vi "Invertor rate calc.vi"(6 "PID gains":T1={"proportional gain (Kc)"=60.0, "integral time (Ti, min)"=0.2, "derivative time (Td, min)"=0.0}, 7 "Output range":cluster{"output high":dbl, "output low":dbl}={"output high"=100.0, "output low"=0.0} {"output low" format="%.2f"; "output high" format="%.2f"}, 9 "V Max Flow":dbl, 10 "process variable g/s":dbl format="%.2f", 11 "User setpoint g/s":dbl format="%.2f") -> (1 "output":dbl format="%.2f", 2 "output V":dbl format="%.2f", 5 "Test Probe":dbl[](array[numeric]))   [LabVIEW 2014]
uses:
  <vilib>/addons/control/pid/pid.llb/PID (DBL).vi
  <vilib>/addons/control/pid/NI_PID_pid.lvlib
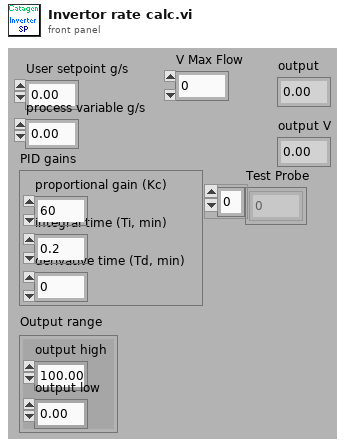
[diagram p1: front panel]
types:
  T1 = cluster{"proportional gain (Kc)":dbl, "integral time (Ti, min)":dbl, "derivative time (Td, min)":dbl}
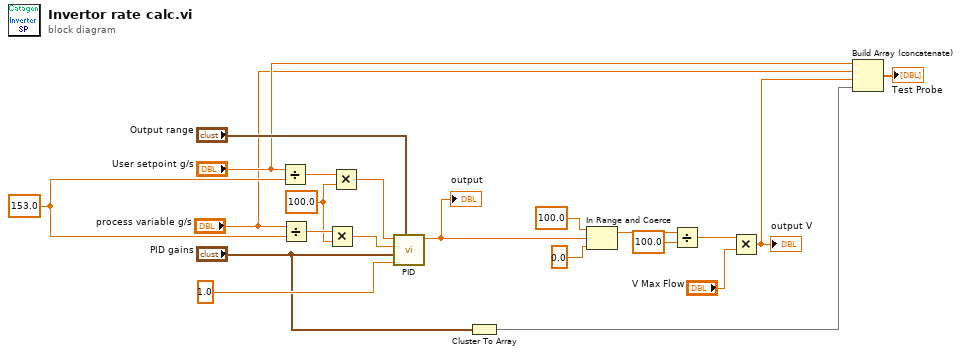
[diagram p0: block diagram]
diagram:
  w8 = 100.0 ("dt (s)")
  w12 = 153.0 ("dt (s)")
  n1 = Divide(x="User setpoint g/s", y=w12) -> (x/y=w11:dbl)
  n2 = Divide(x="process variable g/s", y=w12) -> (x/y=w9:dbl)
  n3 = Multiply(x=w9, y=w8) -> (x*y=w7:dbl)
  n4 = Multiply(x=w11, y=w8) -> (x*y=w10:dbl)
  n5 = call-poly <vilib>:"PID.vi"("output range"="Output range", "dt (s)"=1.0, "PID gains"="PID gains", "process variable"=w7, "setpoint"=w10) -> ("output"=w21:dbl)  [unwired: 5 in, 1 out]
  "output" <- w21
  n6 = Cluster To Array(cluster="PID gains") -> (array=w2:dbl[])
  n7 = In Range and Coerce(upper limit=100.0, x=w21, lower limit=0.0) -> (coerced(x)=w18:dbl)  [unwired: 1 out]
  n8 = Divide(x=w18, y=100.0) -> (x/y=w14:dbl)
  n9 = Multiply(x=w14, y="V Max Flow") -> (x*y=w4:dbl)
  "output V" <- w4
  n10 = Build Array (concatenate)("User setpoint g/s", "process variable g/s", w4, w2) -> (→"Test Probe":dbl[])
